vi "Update GPS data.vi"   [LabVIEW 2010]
uses:
  5.0-Global.vi
types:
  T1 = cluster{"X (Current)":dbl, "Y (Current) ":dbl, "Heading":dbl, "Steering Angle":dbl}
  T2 = typedef "4.2-Where Sensor Typedef.ctl" = cluster{"4.2.2- Current GPS Data":T3, "4.2.1-VectorNav Data":T4, "4.2.1-VectorNav Status":string}
  T3 = typedef "Current GPS Data.ctl" = cluster{"Lattitude (dd.mmmmmm)":ext, "Longitude (dd.mmmmmm)":ext, "EST Time":timestamp}
  T4 = typedef "3.2.1-VectorNav Data.ctl" = cluster{"Yaw":dbl, "Pitch":dbl, "Roll":dbl}
  T5 = cluster{"Lattitude (dd.mmmmmm)":ext, "Longitude (dd.mmmmmm)":ext}
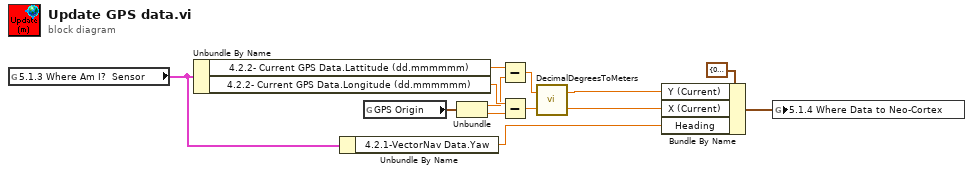
[diagram p0: block diagram]
diagram:
  n1 = global read "5.0-Global.vi" "5.1.3 Where Am I?  Sensor"() -> (w13:T2)
  n2 = Unbundle By Name(w13) -> ("4.2.2- Current GPS Data.Lattitude (dd.mmmmmm)"=w3:ext, "4.2.2- Current GPS Data.Longitude (dd.mmmmmm)"=w5:ext)
  n3 = Unbundle By Name(w13) -> ("4.2.1-VectorNav Data.Yaw"=w12:dbl)
  n4 = global read "5.0-Global.vi" "GPS Origin"() -> (w2:T5)
  n5 = Unbundle(w2) -> ("Lattitude (dd.mmmmmm)"=w4:ext, "Longitude (dd.mmmmmm)"=w6:ext)
  n6 = Subtract(x=w3, y=w4) -> (x-y=w7:ext)
  n7 = Subtract(x=w5, y=w6) -> (x-y=w8:ext)
  n8 = call "DecimalDegreesToMeters.vi"("Longitude"=w8, "Latitude"=w7) -> ("X"=w10:dbl, "Y"=w9:dbl)
  n9 = Bundle By Name(cluster=T1 {"X (Current)"=0.0, "Y (Current) "=0.0, "Heading"=0.0, "Steering Angle"=0.0} ("5.1.4 Where Data to Neo-Cortex"), "Y (Current)"=w9, "X (Current)"=w10, "Heading"=w12) -> (w1:T1)
  n10 = global write "5.0-Global.vi" "5.1.4 Where Data to Neo-Cortex"(w1) -> ()
